vi "Pulse.vi"(2 "error in":errorcluster, 3 "Data in":T1) -> (0 "error out":errorcluster, 1 "Data out":T1)   [LabVIEW 2017, in "Steps.lvlib"]
uses:
  Steps.lvlib
  Type_Defs/Data.ctl
  Type_Defs/Diagnostics.ctl
  Type_Defs/Systems.ctl
panel:
  in  "Step Back":bool
  in  "Continue":bool
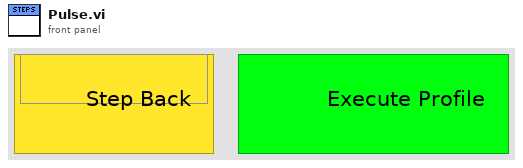
[diagram p1: front panel]
types:
  T1 = typedef "Data.ctl" = cluster{"User Name":string, "Experiment Number":i32, "Start Time":timestamp, "Data":dbl[], "Step Number":i32, "Step Instructions":string, "Diagnostics":T2, "Experiment Purpose":string, "Experiment State":enum16{"Off", "Setting Up", "Ready", "In Progress", "Shutting Down"}, "Systems":T3, "Vacuum Pressure":dbl, "Fieldpoints":cluster{"System Boolean Fieldpoints":cluster{"Compressed Air":refnum<k21>, "T-20kV Power Switch":refnum<k21>, "T-Rectifier":refnum<k21>, "Engage Interlock":refnum<k21>, "Ventilator":refnum<k21>, "Magnetron":refnum<k21>, "H-20kV Power Switch":refnum<k21>, "H-Rectifier":refnum<k21>, "Main Water Pump":refnum<k21>, "WEGA Water Pump":refnum<k21>, "Gas Inlet Valves":refnum<k21>}, "Step Fieldpoints":cluster{"Exhaust Ventillator":refnum<k21>, "Compressed Air":refnum<k21>, "Water Pressure":refnum<k21>, "Interlock":refnum<k21>, "Toroidal Power Supply 1":refnum<k21>, "Toroidal Power Supply 2":refnum<k21>, "Toroidal Rectifier":refnum<k21>, "Helical Power Supply":refnum<k21>, "Helical Rectifier":refnum<k21>, "6kW Magnetron Standby":refnum<k21>, "20kW Magnetron Standby":refnum<k21>}}, "Pressure History":cluster{"Seconds into Experiment":i32[], "Pressure Data":dbl[]}, "Time Computer Control":dbl[], "Toroidal Voltage Computer Control":dbl[], "Helical Voltage Computer Control":dbl[], "Toroidal Current":dbl[], "Toroidal Voltage":dbl[], "Toroidal Current Set Point":dbl[], "Helical Current Set Point":dbl[], "Helical Voltage":dbl[], "Helical Current":dbl[], "Experiment Folder":path, "Run Another Shot?":bool}
  T2 = typedef "Diagnostics.ctl" = cluster{"Langmuir Probe":bool, "Rogowski 1":bool, "Rogowski 2":bool, "Rogowski 3":bool, "B-dot 1":bool, "B-dot 2":bool}
  T3 = typedef "Systems.ctl" = cluster{"Compressed Air":bool, "T-20kV Power Switch":bool, "T-Rectifier":bool, "Engage Interlock":bool, "Ventilator":bool, "Magnetron":bool, "H-20kV Power Switch":bool, "H-Rectifier":bool, "Main Water Pump":bool, "WEGA Water Pump":bool, "Gas Inlet Valves":bool}
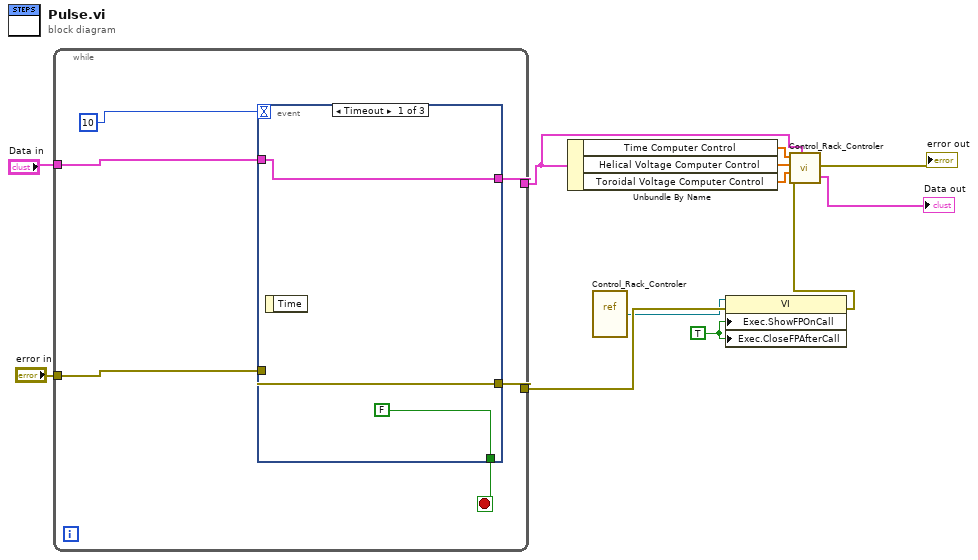
[diagram p0: block diagram]
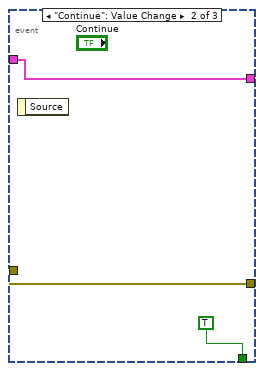
[diagram p2: hidden frame]
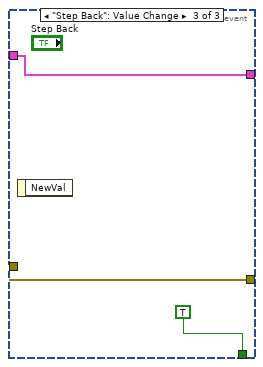
[diagram p3: hidden frame]
diagram:
  w4 = TRUE ("Execution:Show Front Panel On Call")
  n1 = while {
    tunnel: "error in" -> [w18]
    tunnel: [w17] -> w3
    tunnel: [w15] -> w6
    tunnel: "Data in" -> [w14]
    stop <- w16 stop-if-true
    n2 = event shown="[0] Timeout" {
      selector: _ -> [_ _ _]
      dyn-events: _ -> [_ _ _]
      timeout: 10 -> [_ _ _]
      tunnel: w18 -> [w20 w24 w27]
      tunnel: [w20 w24 w27] -> w17
      tunnel: [FALSE TRUE TRUE] -> w16
      tunnel: [w19 w22 w25] -> w15
      tunnel: w14 -> [w19 w22 w25]
      event Timeout {
        n3 = event-data() -> ()  [unwired: 1 in, 1 out]
      }
      event "Continue": Value Change {
        n4 = event-data() -> ()  [unwired: 1 in, 1 out]
      }
      event "Step Back": Value Change {
        n5 = event-data() -> ()  [unwired: 1 in, 1 out]
      }
    }
  }
  n6 = Unbundle By Name(w6) -> ("Time Computer Control"=w9:dbl[], "Helical Voltage Computer Control"=w8:dbl[], "Toroidal Voltage Computer Control"=w7:dbl[])
  n7 = vi-ref "Control_Rack_Controler.vi"() -> (w1:refnum<vi>)
  n8 = property class="VI"(reference=w1, error in=w3, "Exec.ShowFPOnCall"=w4, "Exec.CloseFPAfterCall"=w4) -> (error out=w2:errorcluster)  [unwired: 1 out]
  n9 = call "Control_Rack_Controler.vi"("Times"=w9, "Voltages Toroidal (Keep below |10|)"=w8, "Voltages Helical (Keep below |10|)"=w7, "error out"=w2, "Data out 2"=w6) -> ("error out 2"=→"error out":errorcluster, "Data out"=→"Data out":T1)
